vi "sort 2d array (four columns).vi"(1 "2D array to sort":i32[][](array[numeric])) -> (0 "Sorted array":i32[][](array[numeric]))   [LabVIEW 2015]
doc: "This vi sorts a two-column array in reference to its first column."
panel:
  # "Purpose: This vi sorts a two-column array in reference to its first column."
  # "Instructions: Input a 2D array and then execute the program."
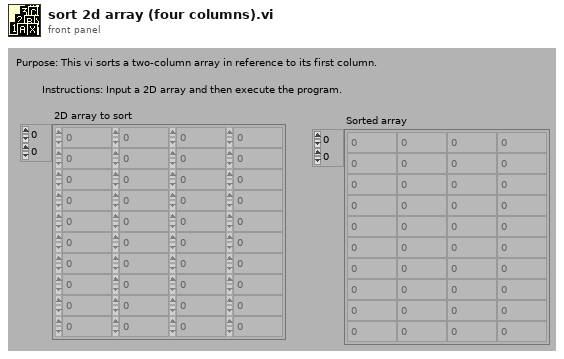
[diagram p1: front panel]
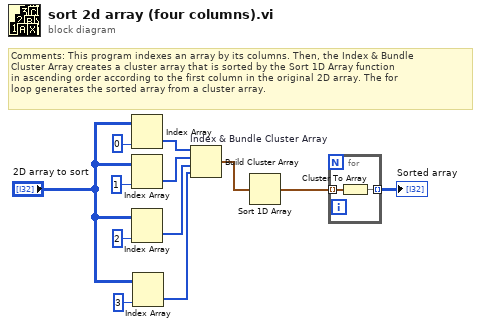
[diagram p0: block diagram]
diagram:
  # "Comments: This program indexes an array by its columns. Then, the Index & Bundle\nCluster Array creates a cluster array that is sorted by the Sort 1D Array function\nin ascending order according to the first column in the original 2D array. The for\nloop generates the sorted array from a cluster array."
  n1 = Index Array(array="2D array to sort", index (col)=0) -> (element=w12:i32[])  [unwired: 1 in]
  n2 = Index Array(array="2D array to sort", index (col)=1) -> (element=w11:i32[])  [unwired: 1 in]
  n3 = Index Array(array="2D array to sort", index (col)=2 ("Disabled Index (col)")) -> (element=w4:i32[])  [unwired: 1 in]
  n4 = Index Array(array="2D array to sort", index (col)=3 ("Disabled Index (col)")) -> (element=w1:i32[])  [unwired: 1 in]
  n5 = Build Cluster Array "Index & Bundle Cluster Array"(w12, w11, w4, w1) -> (w10:cluster{i32, i32, i32, i32}[])
  n6 = Sort 1D Array(array=w10) -> (sorted array=w9:cluster{i32, i32, i32, i32}[])
  n7 = for {
    tunnel: w9 -> [w14] mode=indexing
    tunnel: [w13] -> w8 mode=indexing
    n8 = Cluster To Array(cluster=w14) -> (array=w13:i32[])
  }
  "Sorted array" <- w8
